vi "armCalculator.vi"() -> ()   [LabVIEW 2014]
uses:
  <vilib>/Rock Robotics/WPI/AnalogChannel/WPI_AnalogChannelDevRef.ctl
  <vilib>/Rock Robotics/SystemInterfaces/Typedef/FPGA_TypedefAnalogModule.ctl
  <vilib>/Rock Robotics/SystemInterfaces/AI/FPGA_AIChannel.ctl
  <vilib>/Rock Robotics/WPI/DigitalInput/WPI_DigitalInputDevRef.ctl
  <vilib>/Rock Robotics/SystemInterfaces/DIO/FPGA_DIOChannel.ctl
  <vilib>/Rock Robotics/SystemInterfaces/Typedef/FPGA_TypedefDigitalModule.ctl
panel:
  out "Scaled Pot Val":dbl
  in  "Max Limit Switch":T1={"DevStatus"={"status"=FALSE, "code"=0, "source"=""}, "DIO Channel"=enum."DIO 1", "Controller"=enum."Controller 1"}
  in  "Min Limit Switch":T1={"DevStatus"={"status"=FALSE, "code"=0, "source"=""}, "DIO Channel"=enum."DIO 1", "Controller"=enum."Controller 1"}
  in  "AIDeviceRef":T4={"DevStatus"={"status"=FALSE, "code"=0, "source"=""}, "Controller"=enum."Controller 1", "Analog Channel"=enum."AI 1"}
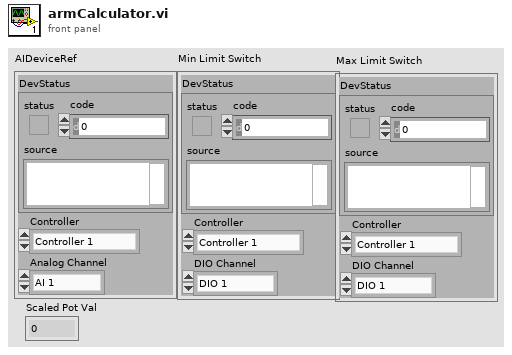
[diagram p1: front panel]
types:
  T1 = typedef "WPI_DigitalInputDevRef.ctl" = cluster{"DevStatus":errorcluster, "DIO Channel":T2, "Controller":T3}
  T2 = typedef "FPGA_DIOChannel.ctl" = enum8{"DIO 0", "DIO 1", "DIO 2", "DIO 3", "DIO 4", "DIO 5", "DIO 6", "DIO 7", "DIO 8", "DIO 9", "DIO MXP 0", "DIO MXP 1", "DIO MXP 2", "DIO MXP 3", "DIO MXP 4", "DIO MXP 5", "DIO MXP 6", "DIO MXP 7", "DIO MXP 8", "DIO MXP 9", "DIO MXP 10", "DIO MXP 11", "DIO MXP 12", "DIO MXP 13", "DIO MXP 14", "DIO MXP 15", "Invalid"}
  T3 = typedef "FPGA_TypedefDigitalModule.ctl" = enum16{"Controller 1"}
  T4 = typedef "WPI_AnalogChannelDevRef.ctl" = cluster{"DevStatus":errorcluster, "Controller":T5, "Analog Channel":T6}
  T5 = typedef "FPGA_TypedefAnalogModule.ctl" = enum16{"Controller 1"}
  T6 = typedef "FPGA_AIChannel.ctl" = enum8{"AI 0", "AI 1", "AI 2", "AI 3", "AI MXP 0", "AI MXP 1", "AI MXP 2", "AI MXP 3", "Invalid"}
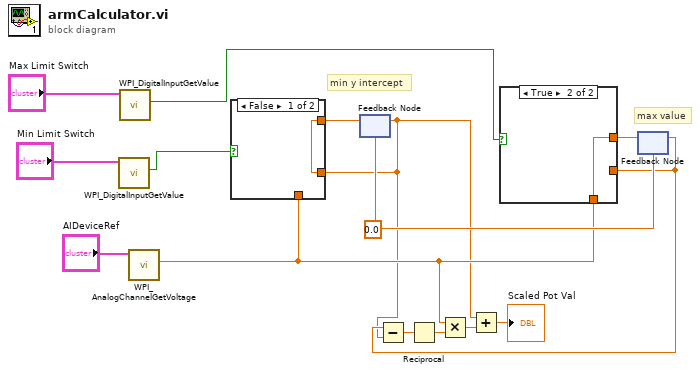
[diagram p0: block diagram]
diagram:
  w10 = 0.0
  # "max value"
  # "min y intercept"
  n1 = call <vilib>:"WPI_DigitalInputGetValue.vi"("DigitalInputDevRef"="Min Limit Switch") -> ("Value"=w12:bool)  [unwired: 8 in, 2 out]
  n2 = call <vilib>:"WPI_DigitalInputGetValue.vi"("DigitalInputDevRef"="Max Limit Switch") -> ("Value"=w9:bool)  [unwired: 8 in, 2 out]
  n3 = call <vilib>:"WPI_AnalogChannelGetVoltage.vi"("AIDeviceRef"="AIDeviceRef") -> ("Voltage"=w7:dbl)  [unwired: 8 in, 2 out]
  n4 = feedback #1(w10) -> (w3:dbl)
  n5 = case shown="False" w12 {
    tunnel: w3 -> [w16 _]
    tunnel: [w16 w17] -> w11
    tunnel: w7 -> [_ w17]
    frame False {
    }
    frame True {
    }
  }
  n6 = feedback-in #1(w11) -> ()
  n7 = feedback #2(w10) -> (w6:dbl)
  n8 = Subtract(x=w6, y=w3) -> (x-y=w5:dbl)
  n9 = Reciprocal(x=w5) -> (1/x=w4:dbl)
  n10 = Multiply(x=w7, y=w4) -> (x*y=w2:dbl)
  n11 = Add(x=w3, y=w2) -> (x+y=→"Scaled Pot Val":dbl)
  n12 = case shown="True" w9 {
    tunnel: [w18 w19] -> w8
    tunnel: w7 -> [_ w19]
    tunnel: w6 -> [w18 _]
    frame False {
    }
    frame True {
    }
  }
  n13 = feedback-in #2(w8) -> ()
